vi "InsertNode.vi"(8 "error in (no error)":errorcluster, 9 "position":T1=enum."Back", 10 "ToInsert":refnum<data-value>, 11 "LLNode in":refnum<class "LLNode.lvclass">) -> (0 "error out":errorcluster, 1 "ignored":bool, 3 "LLNode out":refnum<class "LLNode.lvclass">)   [LabVIEW 2009]
uses:
  Node/Node.lvclass
  LLNode.lvclass
  LinkedList/position.ctl
  LinkedList/LinkedList.lvclass
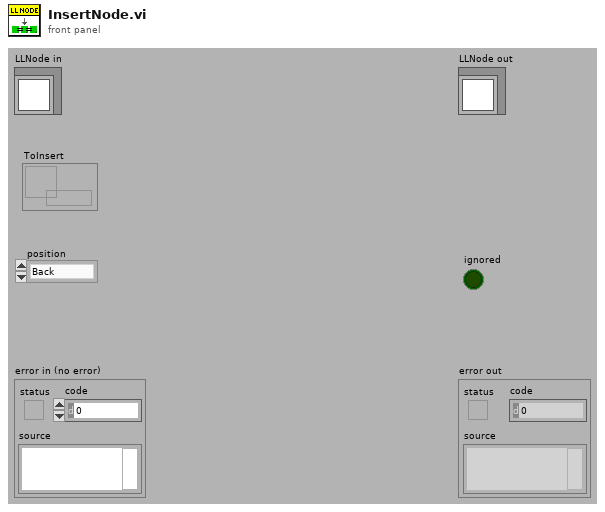
[diagram p1: front panel]
types:
  T1 = typedef "LinkedList.lvclass/position.ctl" = enum16{"Front", "Back", "Search"}
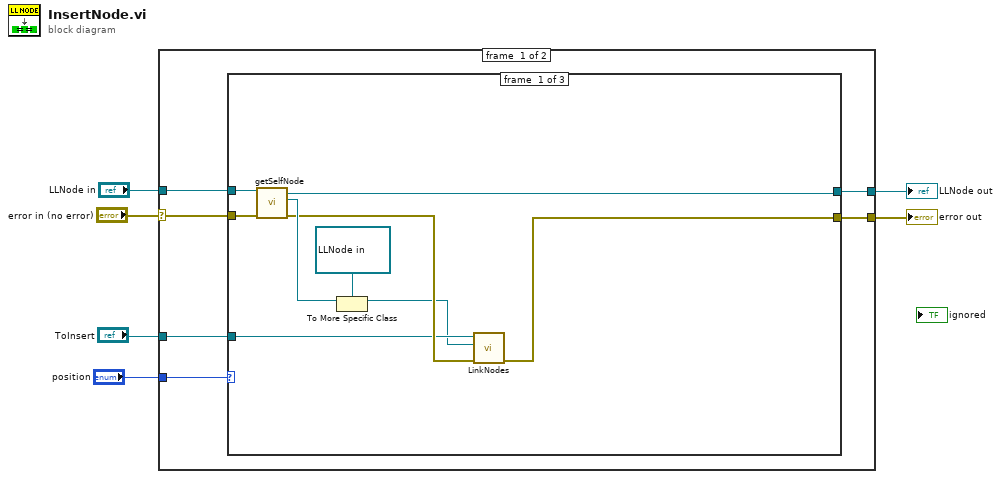
[diagram p0: block diagram]
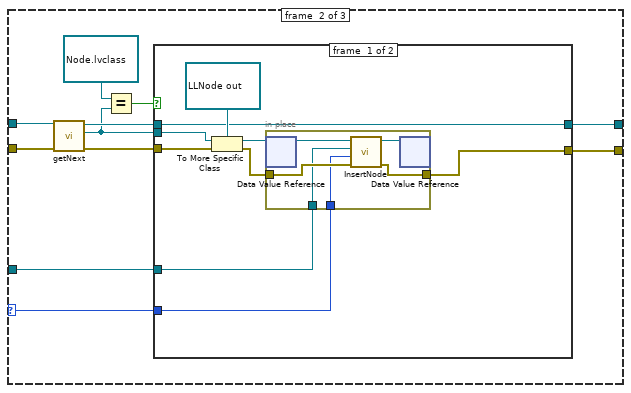
[diagram p2: hidden frame]
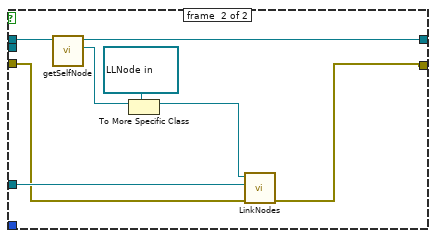
[diagram p3: hidden frame]
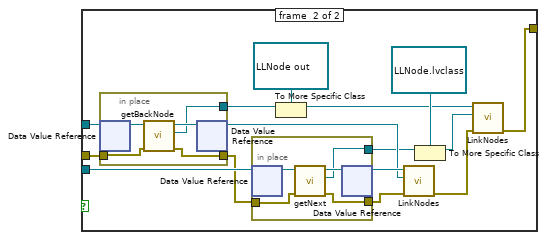
[diagram p5: hidden frame]
diagram:
  n1 = case shown="No Error" "error in (no error)" {
    selector: "error in (no error)" -> [w9 w86]
    tunnel: [w7 w86] -> w5
    tunnel: [w8 w85] -> w4
    tunnel: "LLNode in" -> [w11 w85]
    tunnel: "position" -> [w12 _]
    tunnel: "ToInsert" -> [w10 _]
    frame #0 {
      n2 = case shown="\"Back\"" w12 {
        selector: w12 -> [_ w22 _]
        tunnel: w11 -> [w21 w32 w58]
        tunnel: w10 -> [w15 w26 w57]
        tunnel: w9 -> [w19 w31 w56]
        tunnel: [w17 w25 w58] -> w8
        tunnel: [w13 w24 _] -> w7
        frame #0 {
          n3 = call "getSelfNode.vi"("error in (no error)"=w19, "Node in"=w21) -> ("error out"=w18:errorcluster, "selfNode"=w20:refnum<data-value>, "Node out"=w17:refnum<class "LLNode.lvclass">)  [unwired: 7 in]
          n4 = To More Specific Class(target class=refnum<data-value> refnum ("ToInsert"), reference=w20) -> (specific class reference=w14:refnum<data-value>)  [unwired: 1 in, 1 out]
          n5 = call "LinkNodes.vi"("error in (no error)"=w18, "NextNode in"=w14, "PreviousNode in"=w15) -> ("error out"=w13:errorcluster)  [unwired: 8 in]
        }
        frame #1 {
          n6 = call "getNext.vi"("error in (no error)"=w31, "LLNode in"=w32) -> ("error out"=w28:errorcluster, "next"=w23:refnum<data-value>, "LLNode out"=w27:refnum<class "LLNode.lvclass">)  [unwired: 7 in]
          n7 = Equal?(x=refnum<data-value> refnum, y=w23) -> (x = y?=w29:bool)
          n8 = case shown="False" w29 {
            tunnel: w28 -> [w40 w50]
            tunnel: w27 -> [w36 w55]
            tunnel: w26 -> [w34 w52]
            tunnel: [w36 w49] -> w25
            tunnel: [w35 w48] -> w24
            tunnel: w23 -> [w41 _]
            tunnel: w22 -> [w33 _]
            frame #0 {
              n9 = To More Specific Class(target class=refnum<data-value> refnum ("data value reference"), reference=w41, error in=w40) -> (specific class reference=w38:refnum<data-value>, error out=w37:errorcluster)
              n10 = in-place {
                in-place-border: w37 -> [w46]
                in-place-border: [w45] -> w35
                in-place-border: w34 -> [w43]
                in-place-border: w33 -> [w42]
                n11 = in-place-dvr #1(w38) -> (w44:refnum<class "LLNode.lvclass">)  [unwired: 1 out]
                n12 = call "InsertNode.vi"("error in (no error)"=w46, "position"=w42, "ToInsert"=w43, "LLNode in"=w44) -> ("error out"=w45:errorcluster, "LLNode out"=w47:refnum<class "LLNode.lvclass">)  [unwired: 5 in, 1 out]
                n13 = in-place-dvr #1(w47) -> ()  [unwired: 2 out]
              }
            }
            frame #1 {
              n14 = call "getSelfNode.vi"("Node in"=w55) -> ("selfNode"=w54:refnum<data-value>, "Node out"=w49:refnum<class "LLNode.lvclass">)  [unwired: 8 in, 1 out]
              n15 = To More Specific Class(target class=refnum<data-value> refnum ("data value reference"), reference=w54) -> (specific class reference=w53:refnum<data-value>)  [unwired: 1 in, 1 out]
              n16 = call "LinkNodes.vi"("error in (no error)"=w50, "NextNode in"=w52, "PreviousNode in"=w53) -> ("error out"=w48:errorcluster)  [unwired: 8 in]
            }
          }
        }
        frame #2 {
          n17 = case shown="True" {
            selector: _ -> [_ _]
            tunnel: _ -> [_ w74]
            tunnel: w57 -> [_ w72]
            tunnel: w56 -> [w59 w70]
            tunnel: [w59 w60] -> _
            tunnel: [_ w60] -> _
            frame #0 {
            }
            frame #1 {
              n18 = in-place {
                in-place-border: [w77] -> w69
                in-place-border: w70 -> [w76]
                in-place-border: [w75] -> w63
                n19 = in-place-dvr #2(w72) -> (w79:refnum<class "LLNode.lvclass">)  [unwired: 1 out]
                n20 = call "getBackNode.vi"("error in (no error)"=w76, "LLNode in"=w79) -> ("error out"=w75:errorcluster, "BackNode"=w77:refnum<data-value>, "LLNode out"=w78:refnum<class "LLNode.lvclass">)  [unwired: 7 in]
                n21 = in-place-dvr #2(w78) -> (w71:refnum<data-value>)  [unwired: 1 out]
              }
              n22 = in-place {
                in-place-border: [w82] -> w67
                in-place-border: w63 -> [w81]
                in-place-border: [w80] -> w62
                n23 = in-place-dvr #3(w74) -> (w84:refnum<class "LLNode.lvclass">)  [unwired: 1 out]
                n24 = call "getNext.vi"("error in (no error)"=w81, "LLNode in"=w84) -> ("error out"=w80:errorcluster, "next"=w82:refnum<data-value>, "LLNode out"=w83:refnum<class "LLNode.lvclass">)  [unwired: 7 in]
                n25 = in-place-dvr #3(w83) -> (w73:refnum<data-value>)  [unwired: 1 out]
              }
              n26 = To More Specific Class(target class=refnum<data-value> refnum ("ToInsert"), reference=w69) -> (specific class reference=w65:refnum<data-value>)  [unwired: 1 in, 1 out]
              n27 = call "LinkNodes.vi"("error in (no error)"=w62, "NextNode in"=w71, "PreviousNode in"=w73) -> ("error out"=w61:errorcluster)  [unwired: 8 in]
              n28 = To More Specific Class(target class=refnum<data-value> refnum ("LLNode out"), reference=w67) -> (specific class reference=w64:refnum<data-value>)  [unwired: 1 in, 1 out]
              n29 = call "LinkNodes.vi"("error in (no error)"=w61, "NextNode in"=w64, "PreviousNode in"=w65) -> ("error out"=w60:errorcluster)  [unwired: 8 in]
            }
          }
        }
      }
    }
    frame #1 {
    }
  }
  "error out" <- w5
  "LLNode out" <- w4
